vi "INI Text from JSON.vi"(8 "error in (no error)":errorcluster, 10 "Offset":i32, 11 "Input JSON":string) -> (0 "error out":errorcluster, 1 "Offset after first JSON Value":i32, 3 "Display Text":string)   [LabVIEW 2020, in "JSONtext.lvlib"]
doc: "Reformate JSON as a more human-readable text string, for use in displays. The format is similar to YAML, but may not be fully compliant with that format."
uses:
  <vilib>/JDP Science/JSONtext/JSONtext.lvlib
  <vilib>/JDP Science/JSONtext/Parsing/Advance past Line Ending.vi
  <vilib>/JDP Science/JSONtext/support/quote and escape json string 2.vi
  <vilib>/Utility/error.llb/Error Cluster From Error Code.vi
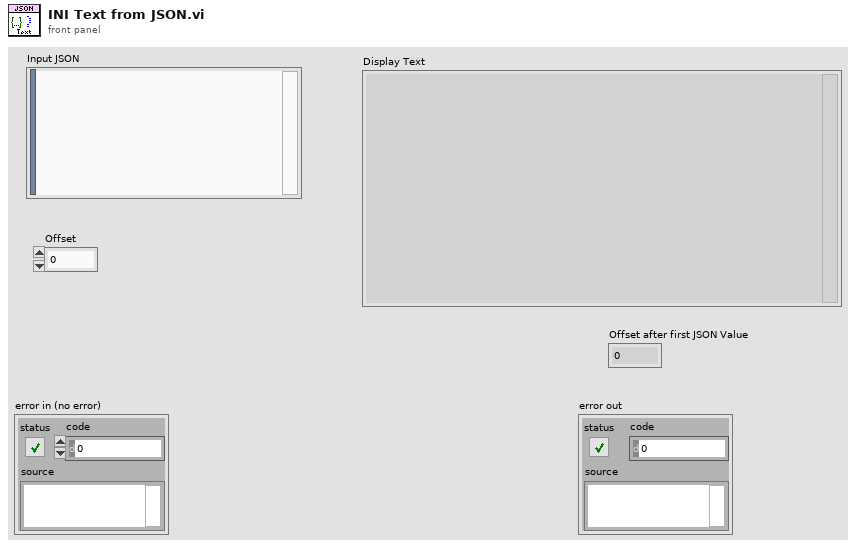
[diagram p1: front panel]
types:
  T1 = typedef "JSONtext.lvlib/Parsing State.ctl" = enum16{"Parser Error", "Object", "Array", "String", "Number/Other", "Leading Whitespace", "Object end", "Array end", "Value end"}
  T2 = typedef "JSONtext.lvlib/JSON Value Type.ctl" = enum16{"Not a JSON Value", "JSON Object", "JSON Array", "String", "Number", "true", "false", "null"}
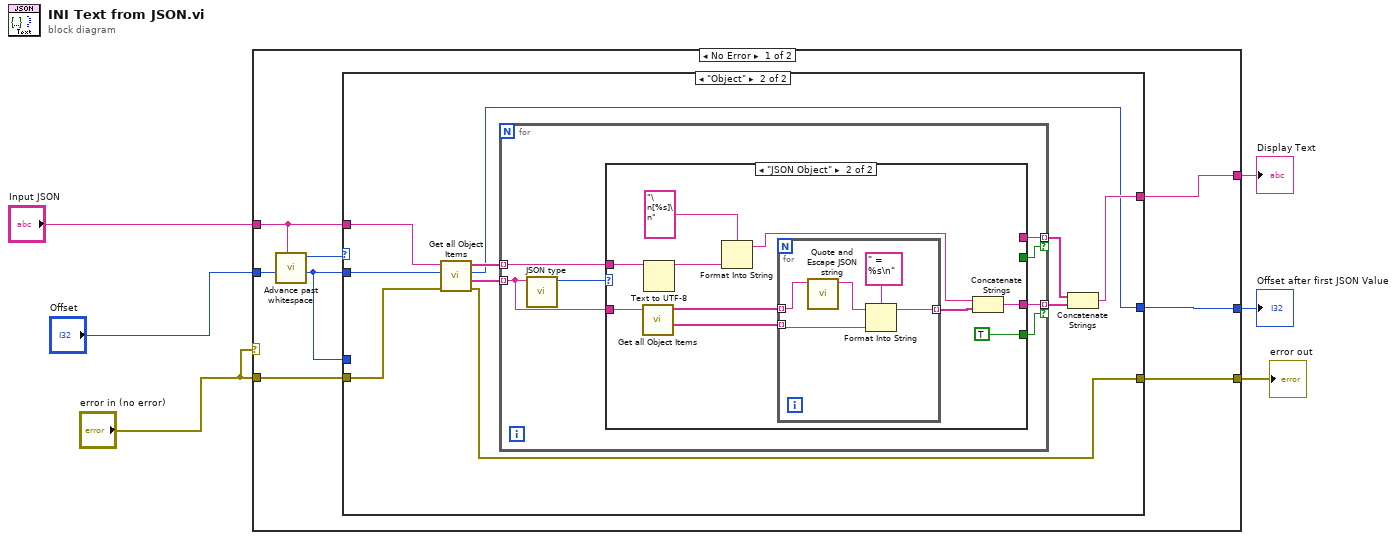
[diagram p0: block diagram]
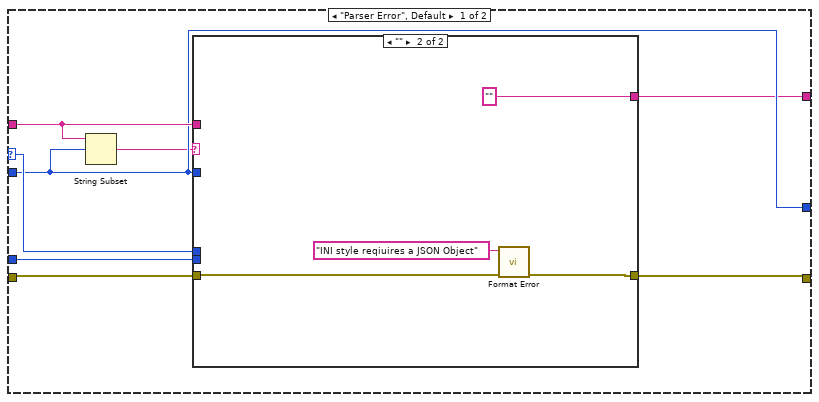
[diagram p2: hidden frame]
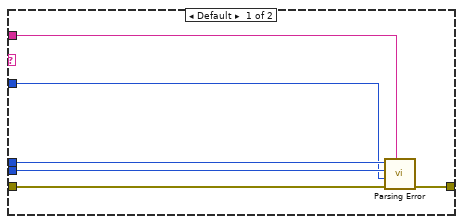
[diagram p3: hidden frame]
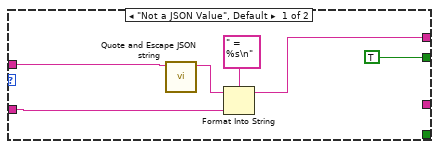
[diagram p4: hidden frame]
diagram:
  n1 = case shown="No Error" "error in (no error)" {
    tunnel: "Input JSON" -> [w14 _]
    tunnel: "Offset" -> [w12 w72]
    tunnel: [w11 w71] -> w4
    tunnel: "error in (no error)" -> [w10 w71]
    tunnel: [w8 _] -> w3
    tunnel: [w7 w72] -> w2
    frame No Error {
      n2 = call <vilib>:"Advance past whitespace.vi"("JSON"=w14, "Offset"=w12) -> ("Offset of first non-whitespace"=w9:i32, "Parser State"=w13:T1)  [unwired: 7 in, 1 out]
      n3 = case shown="\"Object\"" w13 {
        selector: w13 -> [w20 _]
        tunnel: w14 -> [w18 w41]
        tunnel: w9 -> [w17 w42]
        tunnel: [w17 w35] -> w7
        tunnel: [w15 w36] -> w8
        tunnel: [w22 w34] -> w11
        tunnel: w10 -> [w21 w40]
        tunnel: w9 -> [w19 _]
        frame "Parser Error", Default {
          n4 = String Subset(string=w18, offset (0)=w17) -> (substring=w16:string)  [unwired: 1 in]
          n5 = case shown="\"\"" w16 {
            tunnel: [w28 w30] -> w22
            tunnel: w21 -> [w27 w31]
            tunnel: w20 -> [w26 _]
            tunnel: w19 -> [w25 _]
            tunnel: w18 -> [w24 _]
            tunnel: w17 -> [w23 _]
            tunnel: [_ ""] -> w15
            frame Default {
              n6 = call <vilib>:"Parsing Error.vi"("JSON"=w24, "error in (no error)"=w27, "Offset past match"=w23, "Value start"=w25, "State"=w26) -> ("error out"=w28:errorcluster)  [unwired: 6 in]
            }
            frame "" {
              n7 = call <vilib>:"Format Error.vi"("error in (no error)"=w31, "error message"="INI style reqiuires a JSON Object") -> ("error out"=w30:errorcluster)  [unwired: 9 in]
            }
          }
        }
        frame "Object" {
          n8 = call <vilib>:"Get all Object Items.vi"("error in (no error)"=w40, "Offset"=w42, "JSON"=w41) -> ("error out"=w34:errorcluster, "<JSON>"=w39:string[], "Offset past"=w35:i32, "Item Names"=w38:string[])  [unwired: 5 in]
          n9 = for {
            tunnel: w39 -> [w47] mode=indexing
            tunnel: w38 -> [w49] mode=indexing
            tunnel: [w46] -> w37 mode=indexing if=w43
            tunnel: [w45] -> w33 mode=indexing if=w44
            n10 = call <vilib>:"JSON type.vi"("JSON"=w47) -> ("JSON Value Type"=w48:T2)  [unwired: 9 in, 1 out]
            n11 = case shown="\"JSON Object\"" w48 {
              tunnel: w49 -> [w52 w63]
              tunnel: w47 -> [w53 w64]
              tunnel: [_ w57] -> w46
              tunnel: [w51 _] -> w45
              tunnel: [TRUE _] -> w44
              tunnel: [_ TRUE] -> w43
              frame "Not a JSON Value", Default {
                n12 = call <vilib>:"Quote and Escape JSON string.vi"("Plain Text"=w52) -> ("<JSON>"=w55:string)  [unwired: 10 in]
                n13 = Format Into String(format string=" = %s\n", initial string=w55, w53) -> (resulting string=w51:string)  [unwired: 1 in, 1 out]
              }
              frame "JSON Object" {
                n14 = call <vilib>:"Get all Object Items.vi"("JSON"=w64) -> ("<JSON>"=w61:string[], "Item Names"=w60:string[])  [unwired: 7 in, 2 out]
                n15 = Text to UTF-8(11:w63) -> (3:w62:string)  [unwired: 2 in, 1 out]
                n16 = Format Into String(format string="\n[%s]\n", w62) -> (resulting string=w58:string)  [unwired: 2 in, 1 out]
                n17 = for {
                  tunnel: w61 -> [w68] mode=indexing
                  tunnel: w60 -> [w70] mode=indexing
                  tunnel: [w66] -> w59 mode=indexing
                  n18 = call <vilib>:"Quote and Escape JSON string.vi"("Plain Text"=w70) -> ("<JSON>"=w69:string)  [unwired: 10 in]
                  n19 = Format Into String(format string=" = %s\n", initial string=w69, w68) -> (resulting string=w66:string)  [unwired: 1 in, 1 out]
                }
                n20 = Concatenate Strings(w58, w59) -> (w57:string)
              }
            }
          }
          n21 = Concatenate Strings(w33, w37) -> (w36:string)
        }
      }
    }
    frame Error {
    }
  }
  "Offset after first JSON Value" <- w2
  "Display Text" <- w3
  "error out" <- w4
